vi "SensorArray.vi"(0 "Lichteinfallswinkel":dbl(knob)=0.0003312919598386088 scale=-90.0..90.0, 1 "Time s":dbl, 2 "VDD V":dbl=5.0, 3 "Noise Strength":dbl=0.1, 5 "Minimum Angle":i8=-90, 6 "Base Irradiance µW/cm²":dbl=10.0, 9 "Maximum Angle":i8=90, 12 "Gain":dbl=1000.0) -> (4 "Sensor-Gains":dbl[](array[numeric])=[0.044, 0.096, 0.161, 0.256, 0.498, 0.724, 1.098], 10 "Sensor Outputs":dbl[](array[numeric]), 15 "Sensor Frequencies (kHz)":dbl[](array[numeric]))   [LabVIEW 2013]
panel:
  out "Sensor-Gains (Plot)":dbl[](graph)=[0.044, 0.096, 0.161, 0.256, 0.498, 0.724, 1.098]
  # "Osten"
  # "Westen"
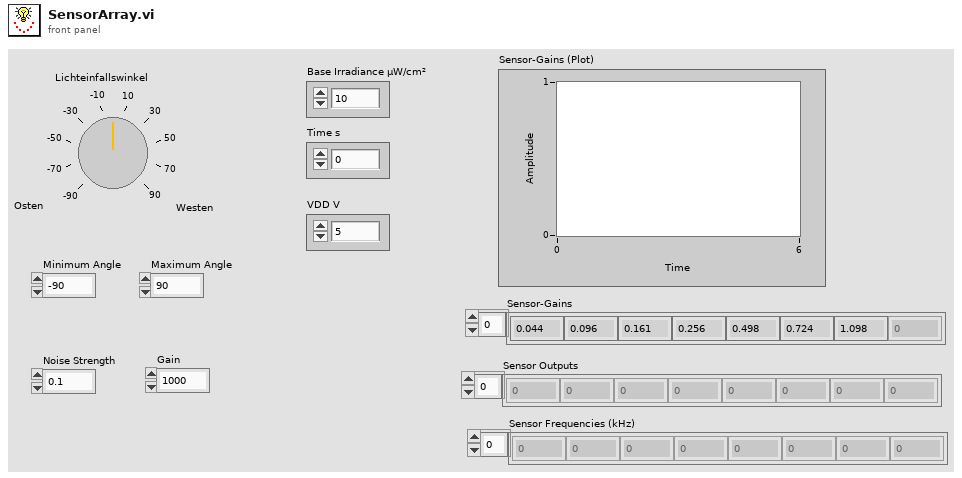
[diagram p1: front panel]
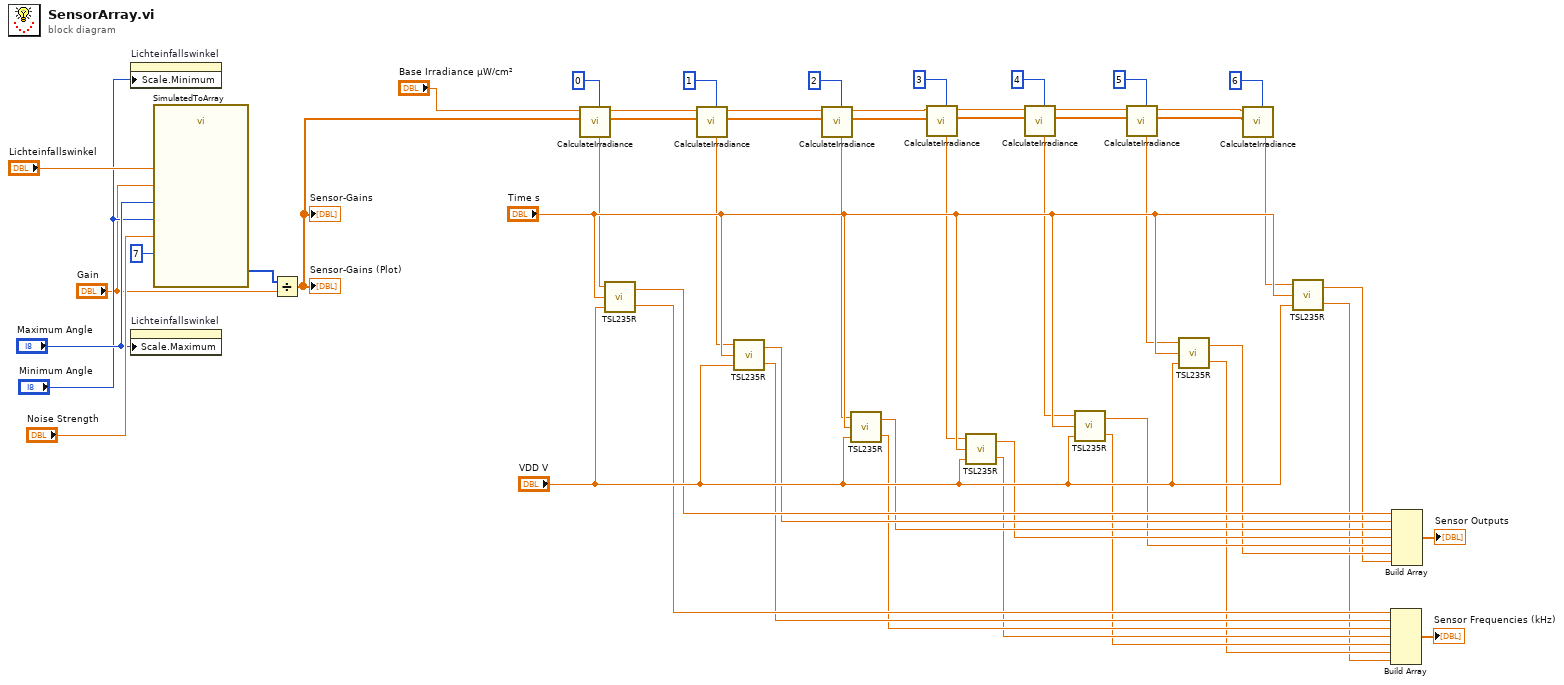
[diagram p0: block diagram]
diagram:
  n1 = property on="Lichteinfallswinkel" class="Knob (strict)"("Scale.Minimum"="Minimum Angle") -> ()  [unwired: 2 in, 2 out]
  n2 = property on="Lichteinfallswinkel" class="Knob (strict)"("Scale.Maximum"="Maximum Angle") -> ()  [unwired: 2 in, 2 out]
  n3 = call "SimulatedToArray.vi"("Gain"="Gain", "Noise Strength"="Noise Strength", "Minimum Angle"="Minimum Angle", "Maximum Angle"="Maximum Angle", "Number of Elements"=u8 7, "Degree"="Lichteinfallswinkel") -> ("Value Array"=w48:u16[])  [unwired: 5 in]
  n4 = Divide(x=w48, y="Gain") -> (x/y=w44:dbl[])
  "Sensor-Gains (Plot)" <- w44
  "Sensor-Gains" <- w44
  n5 = call "CalculateIrradiance.vi"("Base Irradiance µW/cm²"="Base Irradiance µW/cm²", "Array"=w44, "index"=0) -> ("Irradiance"=w39:dbl, "Base Irradiance Out"=w42:dbl, "Array Out"=w41:dbl[])  [unwired: 4 in]
  n6 = call "TSL235R.vi"("VDD V"="VDD V", "Time s"="Time s", "Irradiance µW/cm²"=w39) -> ("Output Frequency (kHz)"=w8:dbl, "Output"=w16:dbl)
  n7 = call "CalculateIrradiance.vi"("Base Irradiance µW/cm²"=w42, "Array"=w41, "index"=1) -> ("Irradiance"=w38:dbl, "Base Irradiance Out"=w22:dbl, "Array Out"=w36:dbl[])  [unwired: 4 in]
  n8 = call "TSL235R.vi"("VDD V"="VDD V", "Time s"="Time s", "Irradiance µW/cm²"=w38) -> ("Output Frequency (kHz)"=w7:dbl, "Output"=w15:dbl)
  n9 = call "CalculateIrradiance.vi"("Base Irradiance µW/cm²"=w22, "Array"=w36, "index"=2) -> ("Irradiance"=w24:dbl, "Base Irradiance Out"=w23:dbl, "Array Out"=w35:dbl[])  [unwired: 4 in]
  n10 = call "TSL235R.vi"("VDD V"="VDD V", "Time s"="Time s", "Irradiance µW/cm²"=w24) -> ("Output Frequency (kHz)"=w6:dbl, "Output"=w14:dbl)
  n11 = call "CalculateIrradiance.vi"("Base Irradiance µW/cm²"=w23, "Array"=w35, "index"=3) -> ("Irradiance"=w28:dbl, "Base Irradiance Out"=w34:dbl, "Array Out"=w33:dbl[])  [unwired: 4 in]
  n12 = call "TSL235R.vi"("VDD V"="VDD V", "Time s"="Time s", "Irradiance µW/cm²"=w28) -> ("Output Frequency (kHz)"=w5:dbl, "Output"=w13:dbl)
  n13 = call "CalculateIrradiance.vi"("Base Irradiance µW/cm²"=w34, "Array"=w33, "index"=4) -> ("Irradiance"=w27:dbl, "Base Irradiance Out"=w32:dbl, "Array Out"=w31:dbl[])  [unwired: 4 in]
  n14 = call "TSL235R.vi"("VDD V"="VDD V", "Time s"="Time s", "Irradiance µW/cm²"=w27) -> ("Output Frequency (kHz)"=w4:dbl, "Output"=w12:dbl)
  n15 = call "CalculateIrradiance.vi"("Base Irradiance µW/cm²"=w32, "Array"=w31, "index"=5) -> ("Irradiance"=w26:dbl, "Base Irradiance Out"=w30:dbl, "Array Out"=w29:dbl[])  [unwired: 4 in]
  n16 = call "TSL235R.vi"("VDD V"="VDD V", "Time s"="Time s", "Irradiance µW/cm²"=w26) -> ("Output Frequency (kHz)"=w3:dbl, "Output"=w11:dbl)
  n17 = call "CalculateIrradiance.vi"("Base Irradiance µW/cm²"=w30, "Array"=w29, "index"=6) -> ("Irradiance"=w25:dbl)  [unwired: 4 in, 2 out]
  n18 = call "TSL235R.vi"("VDD V"="VDD V", "Time s"="Time s", "Irradiance µW/cm²"=w25) -> ("Output Frequency (kHz)"=w2:dbl, "Output"=w10:dbl)
  n19 = Build Array(w8, w7, w6, w5, w4, w3, w2) -> (→"Sensor Frequencies (kHz)":dbl[])
  n20 = Build Array(w16, w15, w14, w13, w12, w11, w10) -> (→"Sensor Outputs":dbl[])
